vi "Create DatabaseTable.vi"() -> ()   [LabVIEW 2018]
doc: "This example allows you to perform several tasks on a database named LabVIEW.mdb located in the LabVIEW examples>>database directory.\n\nOperations include creating a table, creating a table and inserting data into named fields, creating a table and inserting data into generically named fields, or deleting a table."
uses:
  <vilib>/addons/database/Auxilliary.llb/DB Tools Column Info.ctl
  <vilib>/addons/database/Auxilliary.llb/DB Tools DataTypes.ctl
  <vilib>/addons/database/Connection.llb/DB Tools Open Connec (Path).vi
  <vilib>/addons/database/Connection.llb/Conn Execute.vi
  <vilib>/addons/database/Recordset.llb/Rec Fetch Recordset Data (R).vi
  <vilib>/addons/database/NI_Database_API.lvlib
panel:
  out "recordset data":variant[][](array[variant])
  out "columns":string[](array[string])
  out "column information 2":T2(array[cluster])
  in  "connection information":path
  in  "sample data":T3={"String"="This is a test string", "Numeric"=101, "Numeric 2"=3.14}
  in  "column information":T4[](array[typedef])=[{"column name"="stringcol", "data type"=enum."String", "size"=50, "allow null?"=FALSE}, {"column name"="intcol", "data type"=enum."Long (I32)", "size"=0, "allow null?"=TRUE}, {"column name"="doublecol", "data type"=enum."Double (DBL)", "size"=0, "allow null?"=TRUE}]
  in  "Function":u16(ring) items=["Create Only", "Create and Insert (With Names)", "Create and Insert (Generic Names)", "Delete Table", "Get columns", "Insert", "Show data"]
  in  "Table":string="createtable"
  # "Overview: Demonstrates how to perform several tasks on a database.\nRequirements: Database Connectivity Toolkit\nInstructions:\n1. Select one of the 'Create' operations in the Function ring.\n2. Run the VI. The database table will be updated.\n3. Select another 'Create' operation and run the VI again.\n4. Select the 'Delete Table' operation and run the VI to remove the table from the database."
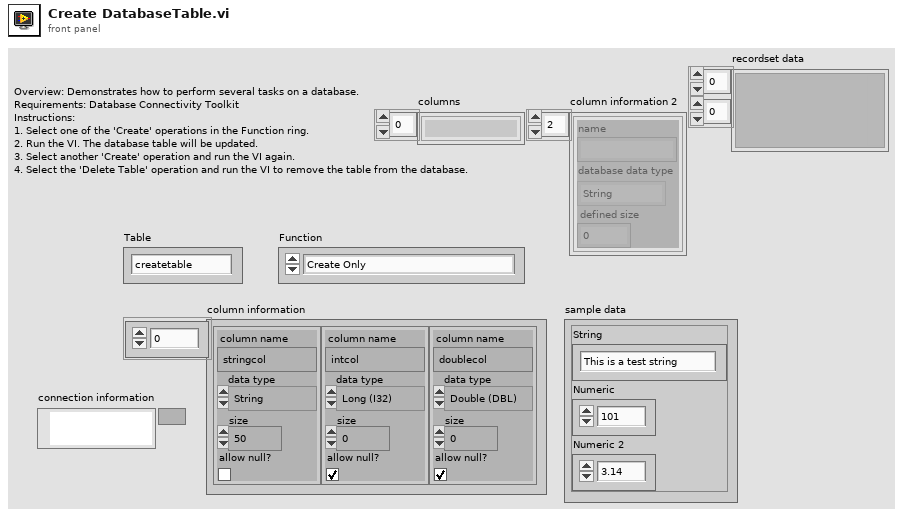
[diagram p1: front panel]
types:
  T1 = typedef "NI_Database_API.lvlib/DB Tools DataTypes.ctl" = enum16{"String", "Long (I32)", "Single (SGL)", "Double (DBL)", "Date/Time", "Binary"}
  T2 = cluster{"name":string, "database data type":T1, "defined size":i32}[]
  T3 = cluster{"String":string, "Numeric":i32, "Numeric 2":dbl}
  T4 = typedef "NI_Database_API.lvlib/DB Tools Column Info.ctl" = cluster{"column name":string, "data type":T1, "size":i32, "allow null?":bool}
  T5 = typedef "NI_Database_API.lvlib/Conn ObjectReference.ctl" = refnum<k1>
  T6 = typedef "NI_Database_API.lvlib/Rec ObjectReference.ctl" = refnum<k1>
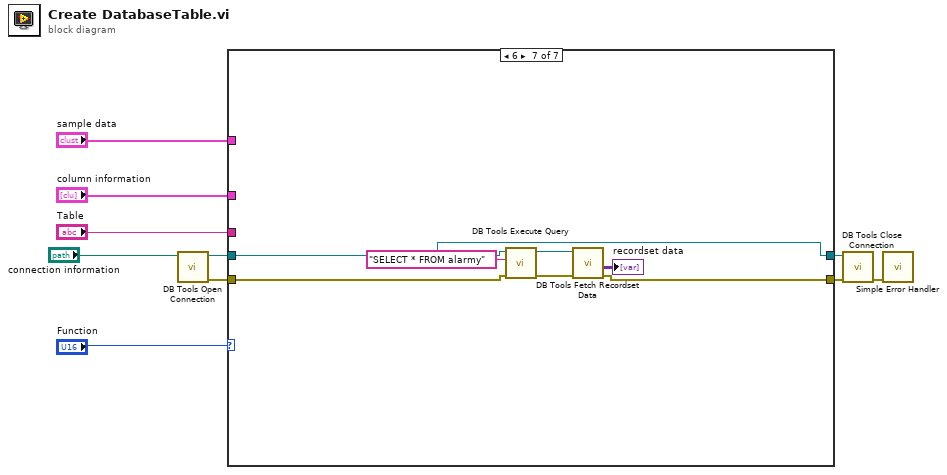
[diagram p0: block diagram]
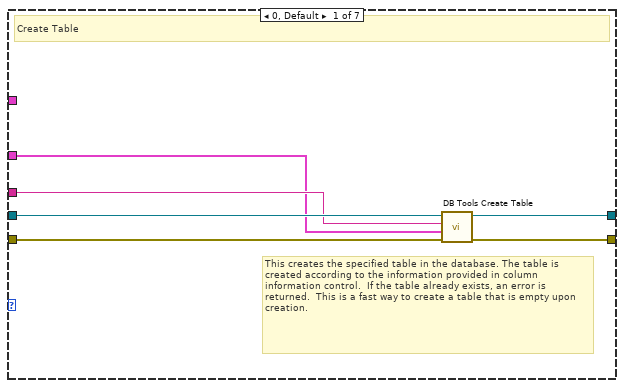
[diagram p2: hidden frame]
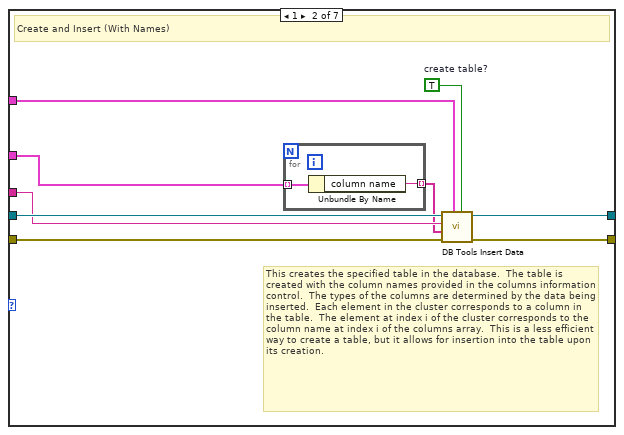
[diagram p3: hidden frame]
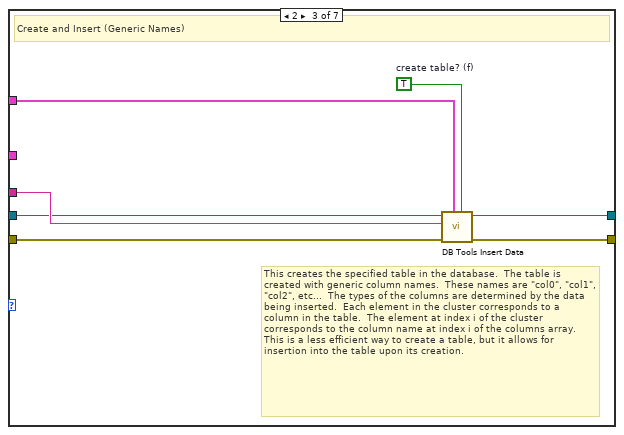
[diagram p4: hidden frame]
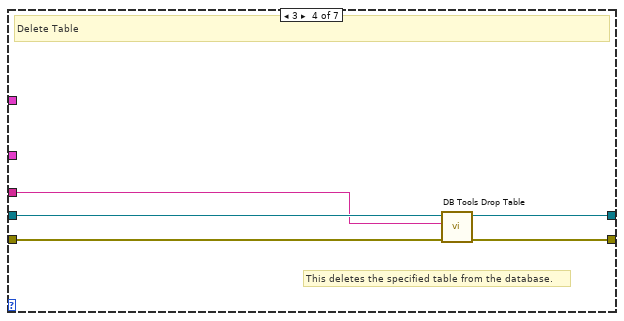
[diagram p5: hidden frame]
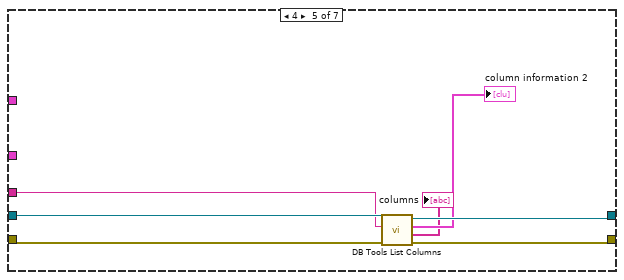
[diagram p6: hidden frame]
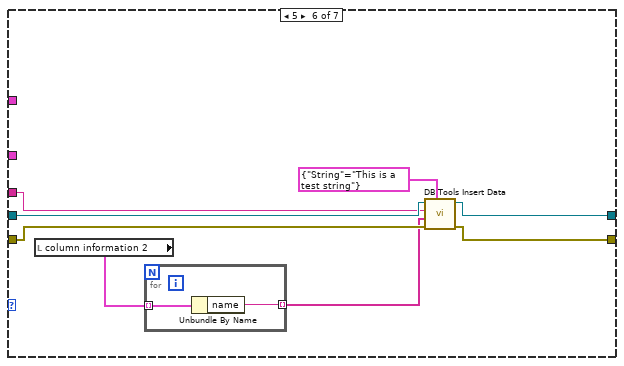
[diagram p7: hidden frame]
diagram:
  n1 = call-poly <vilib>:"DB Tools Open Connection.vi"("connection information"="connection information") -> ("error out"=w6:errorcluster, "connection reference"=w7:T5)  [unwired: 7 in]
  n2 = case shown="6" "Function" {
    tunnel: w7 -> [w16 w25 w29 w39 w46 w54 w57]
    tunnel: w6 -> [w15 w22 w30 w38 w45 w53 w63]
    tunnel: "Table" -> [w14 w19 w31 w35 w42 w49 _]
    tunnel: [w13 w20 w32 w37 w43 w51 w57] -> w9
    tunnel: [w12 w21 w34 w36 w44 w52 w59] -> w8
    tunnel: "sample data" -> [_ w23 w28 _ _ _ _]
    tunnel: "column information" -> [w11 w18 _ _ _ _ _]
    frame 0, Default {
      # "This creates the specified table in the database. The table is created according to the information provided in column information control.  If the table already exists, an error is returned.  This is a fast way to create a table that is empty upon creation."
      # "Create Table"
      n3 = call <vilib>:"DB Tools Create Table.vi"("error in (no error)"=w15, "column information"=w11, "table"=w14, "connection reference"=w16) -> ("error out"=w12:errorcluster, "connection reference out"=w13:T5)  [unwired: 4 in]
    }
    frame 1 {
      w24 = TRUE  # create table?
      # "This creates the specified table in the database.  The table is created with the column names provided in the columns information control.  The types of the columns are determined by the data being inserted.  Each element in the cluster corresponds to a column in the table.  The element at index i of the cluster corresponds to the column name at index i of the columns array.  This is a less efficient way to create a table, but it allows for insertion into the table upon its creation."
      # "Create and Insert (With Names)"
      n4 = for {
        tunnel: w18 -> [w27] mode=indexing
        tunnel: [w26] -> w17 mode=indexing
        n5 = Unbundle By Name(w27) -> ("column name"=w26:string)
      }
      n6 = call <vilib>:"DB Tools Insert Data.vi"("create table? (F)"=w24, "data"=w23, "error in (no error)"=w22, "columns"=w17, "table"=w19, "connection reference"=w25) -> ("error out"=w21:errorcluster, "connection reference out"=w20:T5)  [unwired: 4 in]
    }
    frame 2 {
      w33 = TRUE  # create table? (f)
      # "This creates the specified table in the database.  The table is created with generic column names.  These names are \"col0\", \"col1\", \"col2\", etc...  The types of the columns are determined by the data being inserted.  Each element in the cluster corresponds to a column in the table.  The element at index i of the cluster corresponds to the column name at index i of the columns array.  This is a less efficient way to create a table, but it allows for insertion into the table upon its creation."
      # "Create and Insert (Generic Names)"
      n7 = call <vilib>:"DB Tools Insert Data.vi"("create table? (F)"=w33, "data"=w28, "error in (no error)"=w30, "table"=w31, "connection reference"=w29) -> ("error out"=w34:errorcluster, "connection reference out"=w32:T5)  [unwired: 5 in]
    }
    frame 3 {
      # "This deletes the specified table from the database."
      # "Delete Table"
      n8 = call <vilib>:"DB Tools Drop Table.vi"("error in (no error)"=w38, "table"=w35, "connection reference"=w39) -> ("error out"=w36:errorcluster, "connection reference out"=w37:T5)  [unwired: 5 in]
    }
    frame 4 {
      n9 = call <vilib>:"DB Tools List Columns.vi"("error in (no error)"=w45, "table"=w42, "connection reference"=w46) -> ("error out"=w44:errorcluster, "columns"=→"columns":string[], "column information"=→"column information 2":T2, "connection reference out"=w43:T5)  [unwired: 1 in]
    }
    frame 5 {
      n10 = local read "column information 2"() -> (w48:T2)
      n11 = for {
        tunnel: w48 -> [w56] mode=indexing
        tunnel: [w55] -> w47 mode=indexing
        n12 = Unbundle By Name(w56) -> ("name"=w55:string)
      }
      n13 = call <vilib>:"DB Tools Insert Data.vi"("data"=cluster{"String":string} {"String"="This is a test string"} ("sample data"), "error in (no error)"=w53, "columns"=w47, "table"=w49, "connection reference"=w54) -> ("error out"=w52:errorcluster, "connection reference out"=w51:T5)  [unwired: 5 in]
    }
    frame 6 {
      n14 = call-poly <vilib>:"DB Tools Execute Query.vi"("error in (no error)"=w63, "SQL query"="SELECT * FROM alarmy", "connection reference"=w57) -> ("error out"=w60:errorcluster, "recordset reference"=w61:T6)  [unwired: 5 in]
      n15 = call-poly <vilib>:"DB Tools Fetch Recordset Data.vi"("error in (no error)"=w60, "recordset reference"=w61) -> ("error out"=w59:errorcluster, "recordset data"=→"recordset data":variant[][])  [unwired: 3 in, 1 out]
    }
  }
  n16 = call <vilib>:"DB Tools Close Connection.vi"("error in (no error)"=w8, "connection reference"=w9) -> ("error out"=w4:errorcluster)  [unwired: 5 in]
  n17 = call <vilib>:"Simple Error Handler.vi"("error in (no error)"=w4) -> ()  [unwired: 4 in, 5 out]
